vi "PH_ImageCoG_Plotter.Beam Analysis.vi"(0 "i ref in":refnum<vi>, 5 "error in (no error)":errorcluster) -> (14 "i ref out":refnum<vi>, 19 "error out":errorcluster)   [LabVIEW 2014, in "PH_ImageCoG_Plotter.lvlib"]
doc: "This VI does several beam analysis calculations."
uses:
  PH_ImageCoG_Plotter.lvlib
  PH_Basics/PH_StatusHandler/PH_StatusHandler.Status.ctl
  <vilib>/vision/NI_Vision_Development_Module.lvlib
  PH_Basics/PH_Common/PH_Common.lvlib
  PH_Basics/PH_StatusHandler/PH_StatusHandler.lvlib
panel:
  in  "new element/subarray":T1
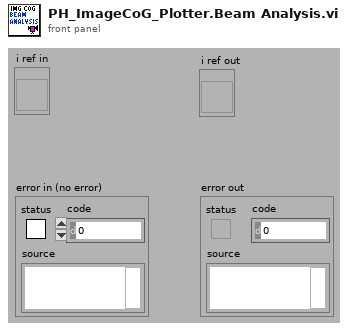
[diagram p1: front panel]
types:
  T1 = cluster{"current time":timestamp, "CoG-x":dbl, "CoG-y":dbl, "Delta-x":dbl, "Delta-y":dbl}
  T2 = typedef "PH_ImageCoG_Plotter.lvlib/PH_ImageCoG_Plotter.i attribute.ctl" = cluster{"GUI Refs":cluster{"Delete":refnum<vi>, "Calibration status":refnum<vi>, "BI subtracted":refnum<vi>, "calc Beam Anal":refnum<vi>, "CoG - x":refnum<vi>, "CoG - y":refnum<vi>, "Type":refnum<vi>, "Center":refnum<vi>, "exp - X":refnum<vi>, "exp - Y":refnum<vi>, "Delta - X":refnum<vi>, "Delta - Y":refnum<vi>, "Available Cams":refnum<vi>, "CoG X":refnum<vi>, "CoG Y":refnum<vi>, "Delta X":refnum<vi>, "Delta Y":refnum<vi>, "Export Data":refnum<vi>, "Calibration data":refnum<vi>}, "Calibration":cluster{"Status":T3, "Calibration data":T4, "Calibration Data File":path}, "Beam Analysis":cluster{"on":bool, "exp - X":i32, "exp - Y":i32, "Type":bool, "Data":cluster{"current time":timestamp, "CoG-x":dbl, "CoG-y":dbl, "Delta-x":dbl, "Delta-y":dbl}[], "Datasets strored":i32, "Dataarray Size":i32}, "Cam instances":string[], "DIM Service Events":T5[], "Images":cluster{"Background":T8, "OP":T8, "GUI":T8}}
  T3 = typedef "PH_StatusHandler.lvlib/PH_StatusHandler.Status.ctl" = i16
  T4 = typedef "PH_ImageCalibrator.lvlib/PH_ImageCalibrator.Calibration Data.ctl" = cluster{"Date":string, "Time":string, "Cam Settings":cluster{"Cam ID":string, "Gain":dbl, "Brightness":dbl, "Shutter":dbl, "Cam Error":bool, "Mode":i32}, "Background Image":cluster{"Image":dbl[][], "Image Error":bool}, "Linear Calibration":cluster{"Calibration Factor":dbl, "not mm or mrad":bool}, "Energy Calibration":cluster{"Calibration Factor":dbl, "no mJ":bool}}
  T5 = typedef "BaseProcess.lvlib/BaseProcess.event definition.ctl" = cluster{"CAEEvtDef":T6, "Data Descriptor":T7}
  T6 = typedef "CAEObj.lvlib/CAEObj.event definition.ctl" = cluster{"URL":string, "enable":bool, "ignoreResID":bool}
  T7 = typedef "BaseProcess.lvlib/BaseProcess.descriptor string definition.ctl" = string
  T8 = typedef "IMAQ Image.ctl" = refnum<image>
  T9 = cluster{"current time":timestamp, "CoG-x":dbl, "CoG-y":dbl, "Delta-x":dbl, "Delta-y":dbl}[]
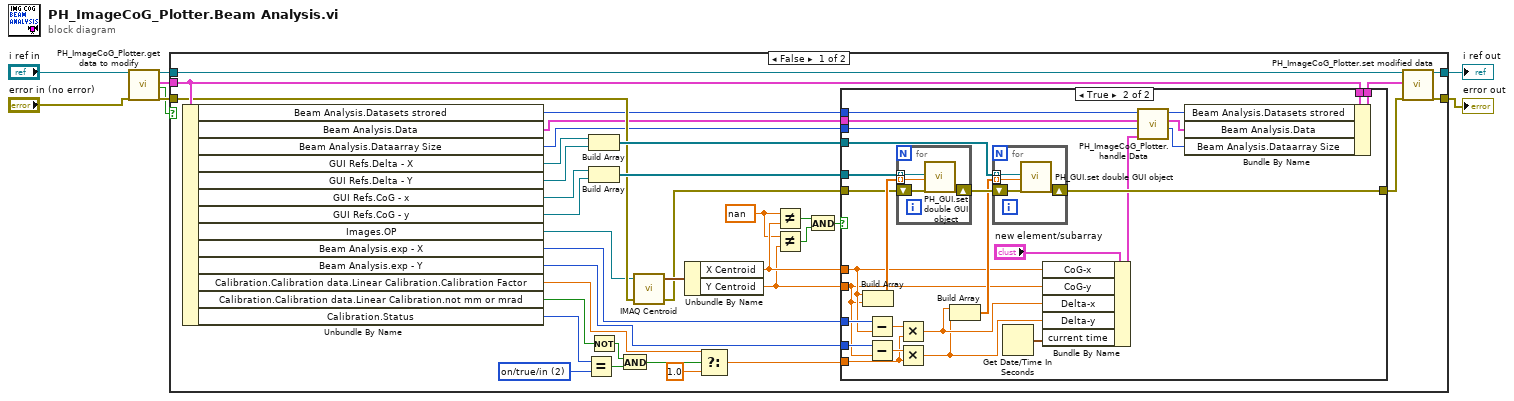
[diagram p0: block diagram]
diagram:
  n1 = call "PH_ImageCoG_Plotter.get data to modify.vi"("i ref in"="i ref in", "error in (no error)"="error in (no error)") -> ("i ref out"=w6:refnum<vi>, "i attribute"=w3:T2, "timed out"=w4:bool, "error out"=w5:errorcluster)  [unwired: 14 in]
  n2 = case shown="False" w4 {
    tunnel: [w36 w82] -> w8
    tunnel: [w35 w83] -> w7
    tunnel: w6 -> [w44 w83]
    tunnel: w5 -> [w30 w82]
    tunnel: w3 -> [w41 _]
    frame False {
      w12 = sgl nan ("x")
      w28 = T3 2 items=["no info", "off/false/out", "on/true/in", "Failure", "Alarm", "Status 1", "Status 2", "Status 3"] ("Calibration.Status")
      n3 = Unbundle By Name(w41) -> ("Beam Analysis.Datasets strored"=w19:i32, "Beam Analysis.Data"=w29:T9, "Beam Analysis.Dataarray Size"=w18:i32, "GUI Refs.Delta - X"=w32:refnum<vi>, "GUI Refs.Delta - Y"=w33:refnum<vi>, "GUI Refs.CoG - x"=w39:refnum<vi>, "GUI Refs.CoG - y"=w38:refnum<vi>, "Images.OP"=w17:T8, "Beam Analysis.exp - X"=w23:i32, "Beam Analysis.exp - Y"=w16:i32, "Calibration.Calibration data.Linear Calibration.Calibration Factor"=w15:dbl, "Calibration.Calibration data.Linear Calibration.not mm or mrad"=w26:bool, "Calibration.Status"=w27:T3)
      n4 = Equal?(x=w27, y=w28) -> (x = y?=w24:bool)
      n5 = Build Array(w32, w33) -> (w31:refnum<vi>[])
      n6 = Build Array(w39, w38) -> (w40:refnum<vi>[])
      n7 = Not(x=w26) -> (.not. x?=w25:bool)
      n8 = And(x=w25, y=w24) -> (x .and. y?=w22:bool)
      n9 = call "IMAQ Centroid"("error in (no error)"=w30, "Image"=w17) -> ("error out"=w37:errorcluster, "Centroid"=w42:cluster{"X Centroid":sgl, "Y Centroid":sgl})  [unwired: 2 in]
      n10 = Unbundle By Name(w42) -> ("X Centroid"=w14:sgl, "Y Centroid"=w13:sgl)
      n11 = Select(t=w15, s=w22, f=1.0) -> (s? t:f=w21:dbl)
      n12 = Not Equal?(x=w12, y=w14) -> (x != y?=w11:bool)
      n13 = Not Equal?(x=w12, y=w13) -> (x != y?=w10:bool)
      n14 = And(x=w11, y=w10) -> (x .and. y?=w9:bool)
      n15 = case shown="True" w9 {
        tunnel: [w45 w73] -> w43
        tunnel: w41 -> [w45 w72]
        tunnel: w40 -> [_ w69]
        tunnel: w37 -> [w46 w68]
        tunnel: [w46 w66] -> w34
        tunnel: w31 -> [_ w65]
        tunnel: w29 -> [_ w59]
        tunnel: w23 -> [_ w55]
        tunnel: w21 -> [_ w54]
        tunnel: w19 -> [_ w51]
        tunnel: w18 -> [_ w50]
        tunnel: w16 -> [_ w49]
        tunnel: w14 -> [_ w48]
        tunnel: w13 -> [_ w47]
        frame False {
        }
        frame True {
          n16 = Build Array(w48, w47) -> (w70:sgl[])
          n17 = Subtract(x=w55, y=w48) -> (x-y=w64:sgl)
          n18 = Subtract(x=w49, y=w47) -> (x-y=w63:sgl)
          n19 = for "Dig Elements" {
            tunnel: w69 -> [w79] mode=indexing
            shift-right: [w80] -> w67
            shift-left: w68 -> [w81]
            tunnel: w70 -> [w78] mode=indexing
            n20 = call "PH_GUI.set double GUI object.vi"("GUI object Ref"=w79, "value"=w78, "error in (no error)"=w81) -> ("error out"=w80:errorcluster)  [unwired: 16 in]
          }
          n21 = Multiply(x=w64, y=w54) -> (x*y=w58:dbl)
          n22 = Multiply(x=w63, y=w54) -> (x*y=w56:dbl)
          n23 = Build Array(w58, w56) -> (w57:dbl[])
          n24 = for "Dig Elements" {
            tunnel: w65 -> [w75] mode=indexing
            shift-right: [w76] -> w66
            shift-left: w67 -> [w77]
            tunnel: w57 -> [w74] mode=indexing
            n25 = call "PH_GUI.set double GUI object.vi"("GUI object Ref"=w75, "value"=w74, "error in (no error)"=w77) -> ("error out"=w76:errorcluster)  [unwired: 16 in]
          }
          n26 = Get Date/Time In Seconds() -> (seconds since 1Jan1904=w60:timestamp)
          n27 = Bundle By Name(cluster="new element/subarray", "CoG-x"=w48, "CoG-y"=w47, "Delta-x"=w58, "Delta-y"=w56, "current time"=w60) -> (w61:T1)
          n28 = call "PH_ImageCoG_Plotter.handle Data.vi"("new Dataset"=w61, "Dataarray Size in"=w50, "Data in"=w59, "Datasets strored in"=w51) -> ("Dataarray Size out"=w52:i32, "Data Out"=w71:T9, "Datasets strored out"=w53:i32)  [unwired: 3 in]
          n29 = Bundle By Name(cluster=w72, "Beam Analysis.Datasets strored"=w53, "Beam Analysis.Data"=w71, "Beam Analysis.Dataarray Size"=w52) -> (w73:T2)
        }
      }
      n30 = call "PH_ImageCoG_Plotter.set modified data.vi"("i ref in"=w44, "i attribute"=w43, "error in (no error)"=w34) -> ("i ref out"=w35:refnum<vi>, "error out"=w36:errorcluster)  [unwired: 15 in]
    }
    frame True {
    }
  }
  "error out" <- w8
  "i ref out" <- w7
